vi "ProcessPoint.vi"(9 "X":dbl, 10 "Y":dbl, 11 "Array in":dbl[][][](array[numeric])) -> (2 "Array out":dbl[][][](array[numeric]), 3 "SceneObject out":refnum<vi>)   [LabVIEW 2018]
uses:
  <vilib>/Analysis/Matrix/Datatypes/RealMatrix.ctl
  <vilib>/Analysis/Matrix/NI_Matrix.lvlib
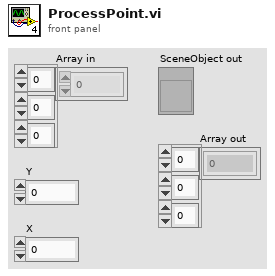
[diagram p1: front panel]
types:
  T1 = cluster{"Line width":sgl, "Line Color":u32, "Axes?":bool}
  T2 = typedef "NI_Matrix.lvlib/RealMatrix.ctl" = dbl[][]
  T3 = cluster{"Theta":dbl, "d":dbl, "a":dbl, "alpha (degrees)":dbl}[]
  T4 = cluster{"Theta":dbl, "d":dbl, "a":dbl, "alpha (degrees)":dbl}
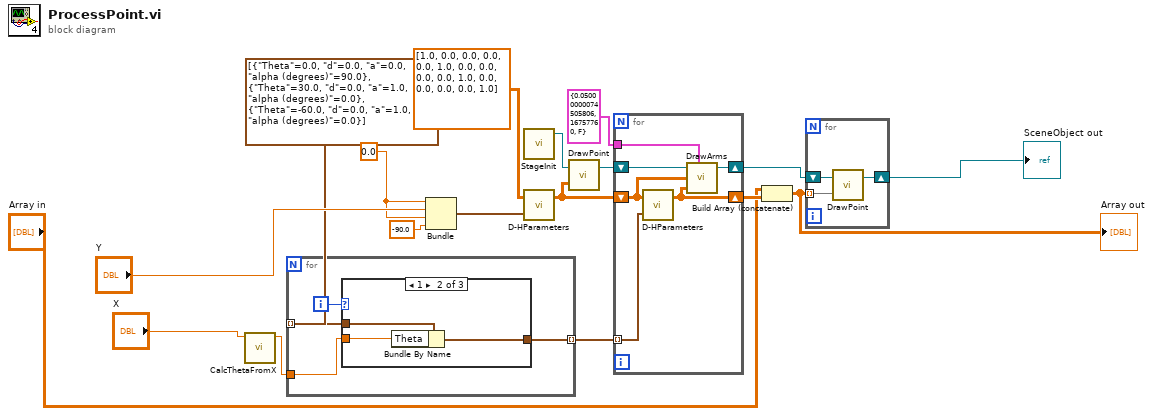
[diagram p0: block diagram]
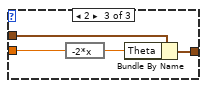
[diagram p3: hidden frame]
diagram:
  w15 = 0.0
  n1 = call "CalcThetaFromX.vi"("X"="X") -> ("Numeric"=w18:dbl)  [unwired: 10 in]
  n2 = for {
    tunnel: T3 [{"Theta"=0.0, "d"=0.0, "a"=0.0, "alpha (degrees)"=90.0}, {"Theta"=30.0, "d"=0.0, "a"=1.0, "alpha (degrees)"=0.0}, {"Theta"=-60.0, "d"=0.0, "a"=1.0, "alpha (degrees)"=0.0}] ("Joints") -> [w21] mode=indexing
    tunnel: [w20] -> w6 mode=indexing
    tunnel: w18 -> [w19]
    i -> [w22]
    n3 = case shown="1" w22 {
      tunnel: w21 -> [w23 w26 w30]
      tunnel: [w23 w25 w29] -> w20
      tunnel: w19 -> [_ w24 w28]
      frame 0, Default {
      }
      frame 1 {
        n4 = Bundle By Name(cluster=w26, "Theta"=w24) -> (w25:T4)
      }
      frame 2 {
        n5 = expression code="-2*x"(w28) -> (w27:dbl)
        n6 = Bundle By Name(cluster=w30, "Theta"=w27) -> (w29:T4)
      }
    }
  }
  n7 = Bundle(w15, "Y"="Y", w15, -90.0) -> (w14:cluster{dbl, "Y":dbl, dbl, dbl})  [unwired: 1 in]
  n8 = call "StageInit.vi"() -> ("Stage out"=w9:refnum<vi>)  [unwired: 4 in, 1 out]
  n9 = call "D-HParameters.vi"("n+1"=w14, "Start"=T2 [[1.0, 0.0, 0.0, 0.0], [0.0, 1.0, 0.0, 0.0], [0.0, 0.0, 1.0, 0.0], [0.0, 0.0, 0.0, 1.0]]) -> ("A x B"=w12:T2)  [unwired: 1 in]
  n10 = call "DrawPoint.vi"("Start"=w12, "Stage in"=w9) -> ("Stage out"=w10:refnum<vi>)  [unwired: 1 in]
  n11 = for {
    shift-right: [w31] -> w5
    shift-left: w12 -> [w32]
    tunnel: w6 -> [w36] mode=indexing
    shift-right: [w34] -> w7
    shift-left: w10 -> [w33]
    tunnel: T1 {"Line width"=0.05, "Line Color"=16757760, "Axes?"=FALSE} ("Params") -> [w35]
    n12 = call "D-HParameters.vi"("n+1"=w36, "Start"=w32) -> ("A x B"=w31:T2)  [unwired: 1 in]
    n13 = call "DrawArms.vi"("Stage in"=w33, "Params"=w35, "Start"=w32, "End"=w31) -> ("Stage out"=w34:refnum<vi>)  [unwired: 2 in, 1 out]
  }
  n14 = Build Array (concatenate)("Array in", w5) -> (w2:dbl[][][])
  "Array out" <- w2
  n15 = for {
    shift-right: [w38] -> w3
    shift-left: w7 -> [w39]
    tunnel: w2 -> [w37] mode=indexing
    n16 = call "DrawPoint.vi"("Start"=w37, "Stage in"=w39) -> ("Stage out"=w38:refnum<vi>)  [unwired: 1 in]
  }
  "SceneObject out" <- w3
